vi "UHR-Fleezers Control (host) - 12.6.vi"() -> ()   [LabVIEW 2012] (continued)
          frame #0 {
            n636 = property on="Saved AOD Raster Scan Parameter Sets" class="Arr (strict)"("Index Values"=u32[] [1]) -> ()  [unwired: 2 in, 2 out]
          }
          frame #1 {
            n637 = Multiply(x="N Steps", y="Step Size (nm)") -> (x*y=w1003:dbl)
            n638 = property on="Scan Speed AOD (nm/s) 2" class="DigNum (strict)"("Value"="Step Size (nm)") -> ()  [unwired: 2 in, 2 out]
            n639 = property on="Step Size AOD (nm) 2" class="DigNum (strict)"("Value"="Step Size (nm)") -> ()  [unwired: 2 in, 2 out]
            n640 = property on="Scan Range AOD (nm) 2" class="DigNum (strict)"("Value"=w1003) -> ()  [unwired: 2 in, 2 out]
          }
        }
      }
      event "Take Detection Laser\nImage": Value Change {
        n641 = event-data() -> ()  [unwired: 1 in, 5 out]
        n642 = flat-sequence {
          tunnel: [w1031] -> w1021
          tunnel: [w1030] -> w1014
          tunnel: [w1029] -> w1006
          tunnel: [w1034] -> w1022
          tunnel: w1021 -> [w1034]
          tunnel: [w1033] -> w1015
          tunnel: w1014 -> [w1033]
          tunnel: [w1032] -> w1007
          tunnel: w1006 -> [w1032]
          tunnel: [w1038] -> w1023
          tunnel: w1022 -> [w1038]
          tunnel: [w1037] -> w1016
          tunnel: w1015 -> [w1037]
          tunnel: [w1036] -> w1008
          tunnel: w1007 -> [w1036]
          tunnel: [w1044] -> w1024
          tunnel: w1023 -> [w1044]
          tunnel: [w1043] -> w1017
          tunnel: w1016 -> [w1043]
          tunnel: [w1042] -> w1009
          tunnel: w1008 -> [w1042]
          tunnel: [w1048] -> w1025
          tunnel: w1024 -> [w1048]
          tunnel: [w1047] -> w1018
          tunnel: w1017 -> [w1047]
          tunnel: [w1046] -> w1010
          tunnel: w1009 -> [w1046]
          tunnel: [w1052] -> w1026
          tunnel: w1025 -> [w1052]
          tunnel: [w1051] -> w1019
          tunnel: w1018 -> [w1051]
          tunnel: [w1050] -> w1011
          tunnel: w1010 -> [w1050]
          tunnel: [w1056] -> w1027
          tunnel: w1026 -> [w1056]
          tunnel: [w1055] -> w1020
          tunnel: w1019 -> [w1055]
          tunnel: [w1054] -> w1012
          tunnel: w1011 -> [w1054]
          tunnel: w1027 -> [w1062]
          tunnel: w1020 -> [w1061]
          tunnel: [w1059] -> w1013
          tunnel: w1012 -> [w1059]
          tunnel: w1013 -> [w1063]
          frame #0 {
            n643 = local read "Laser interlacing mode"() -> (w1030:enum32{"Laser ON", "Laser OFF", "Interlace"})
            n644 = local read "Green FB On/Off"() -> (w1029:bool)
            n645 = local read "Green Laser ON"() -> (w1031:bool)
          }
          frame #1 {
            n646 = property on="Green FB On/Off" class="Bool (strict)"("Val(Sgnl)"=FALSE ("Value (Signaling)")) -> ()  [unwired: 2 in, 2 out]
          }
          frame #2 {
            n647 = property on="Green Laser ON" class="Bool (strict)"("Val(Sgnl)"=TRUE ("Value (Signaling)")) -> ()  [unwired: 2 in, 2 out]
            n648 = property on="Flip Green Filter" class="Bool (strict)"("Val(Sgnl)"=TRUE ("Value (Signaling)")) -> ()  [unwired: 2 in, 2 out]
            n649 = property on="Laser interlacing mode" class="RadioBtnsControl (strict)"("Val(Sgnl)"=enum32{"Laser ON", "Laser OFF", "Interlace"}."Laser ON" ("Value (Signaling)")) -> ()  [unwired: 2 in, 2 out]
          }
          frame #3 {
            n650 = Wait (ms)(milliseconds to wait=u32 500) -> ()  [unwired: 1 out]
          }
          frame #4 {
            n651 = property on="Confocal Image" class="Bool (strict)"("Val(Sgnl)"=TRUE ("Value (Signaling)")) -> ()  [unwired: 2 in, 2 out]
          }
          frame #5 {
            n652 = Wait (ms)(milliseconds to wait=u32 2000) -> ()  [unwired: 1 out]
          }
          frame #6 {
            n653 = while {
              stop <- w1057 stop-if-true
              n654 = local read "Saving..."() -> (w1058:bool)
              n655 = Not(x=w1058) -> (.not. x?=w1057:bool)
            }
          }
          frame #7 {
            n656 = property on="Flip Green Filter" class="Bool (strict)"("Val(Sgnl)"=TRUE ("Value (Signaling)")) -> ()  [unwired: 2 in, 2 out]
            n657 = property on="Green Laser ON" class="Bool (strict)"("Val(Sgnl)"=w1062) -> ()  [unwired: 2 in, 2 out]
            n658 = property on="Laser interlacing mode" class="RadioBtnsControl (strict)"("Val(Sgnl)"=w1061) -> ()  [unwired: 2 in, 2 out]
          }
          frame #8 {
            n659 = property on="Green FB On/Off" class="Bool (strict)"("Val(Sgnl)"=w1063) -> ()  [unwired: 2 in, 2 out]
          }
        }
      }
      event "Stop All": Value Change {
        # "Stopping blue laser before shutting off program"
        n660 = event-data() -> ()  [unwired: 1 in, 5 out]
        n661 = local read "Delay (ms)"() -> (w1066:i32)
        n662 = call "serial write macro.vi"("String"="l0", "Delay (ms)"=w1066, "VISA resource name"=w1069) -> ("read buffer"=w1064:string, "error out"=w1065:errorcluster, "VISA resource name out"=w1068:refnum<visa-resource-name>)
        n663 = local write "read blue buffer"(w1064) -> ()
        n664 = local write "Blue Error Out"(w1065) -> ()
        n665 = VISA Close(VISA resource name=w1068) -> ()  [unwired: 1 in, 1 out]
        n666 = local read "Stop All"() -> (w1070:bool)
      }
    }
    n667 = node-c288() -> ()  [unwired: 1 in, 1 out]
  }
  n668 = node-c288() -> (w10:T23)  [unwired: 4 out]
  n669 = timed-loop "Oscillate Trap/AOM (fishing, conjugate plane alignment)" {
    tunnel: w16 -> [w1072]
    tunnel: [w1071] -> w129
    timing: w124 -> [_]
    timing-out: [_] -> w123
    stop <- w1071 stop-if-true
    n670 = node-c288() -> ()  [unwired: 2 out]
    n671 = event shown="[0] \"Oscillate Set 1\", \"Fish for Tether\": Value Change" {
      selector: _ -> [_ _ _]
      dyn-events: _ -> [_ _ _]
      timeout: _ -> [_ _ _]
      tunnel: w1072 -> [w1079 _ _]
      tunnel: [FALSE ("Stop All") _ w1677] -> w1071
      event "Oscillate Set 1", "Fish for Tether": Value Change {
        n672 = event-data() -> ()  [unwired: 6 out]
        n673 = local read "Oscillate Set 1"() -> (w1078:bool)
        n674 = Or(x=w1078, y="Fish for Tether") -> (x .or. y?=w1076:bool)
        n675 = case shown="True" w1076 {
          tunnel: w1079 -> [_ w1082]
          tunnel: "Fish for Tether" -> [_ w1081]
          frame False {
          }
          frame True {
            n676 = case shown="True" w1081 {
              selector: w1081 -> [w1085 w1091]
              tunnel: [w1085 w1091] -> w1080
              frame False {
              }
              frame True {
                n677 = local write "Scan axis 2"(TRUE) -> ()
                n678 = local write "Tether"(FALSE ("Tether")) -> ()
                n679 = local read "Flow ON during cal?"() -> (w1086:bool)
                n680 = property on="Trap Delta (MHz)" class="DigNum (strict)"("Val(Sgnl)"="Furthest Delta (MHz)") -> ()  [unwired: 2 in, 2 out]
                n681 = Or(x="Flow ON during \nfishing?", y=w1086) -> (x .or. y?=w1087:bool)
                n682 = Wait (ms)(milliseconds to wait=u32 500) -> ()  [unwired: 1 out]
                n683 = property on="Sample Channel\nFlow" class="Bool (strict)"("Val(Sgnl)"=w1087) -> ()  [unwired: 2 in, 2 out]
              }
            }
            n684 = node-c288() -> (w1084:T23)  [unwired: 1 in, 3 out]
            n685 = timed-loop "Oscillate AOD" {
              timing: w1084 -> [_]
              timing-out: [_] -> w1083
              tunnel: w1082 -> [w1101]
              tunnel: w1080 -> [w1094]
              i -> [w1103]
              stop <- w1100 stop-if-true
              n686 = node-c288() -> (w1102:i64)  [unwired: 1 out]
              n687 = flat-sequence {
                tunnel: w1103 -> [w1130]
                tunnel: w1102 -> [w1129]
                tunnel: w1101 -> [w1111]
                tunnel: w1094 -> [w1113]
                tunnel: [w1113] -> w1099
                tunnel: [w1112] -> w1098
                tunnel: [w1110] -> w1097
                tunnel: [w1107] -> w1095
                tunnel: w1099 -> [w1175]
                tunnel: w1098 -> [w1173]
                tunnel: w1097 -> [w1172]
                tunnel: [w1171] -> w1096
                tunnel: w1095 -> [w1170]
                tunnel: [w1247] -> w1100
                tunnel: w1096 -> [w1246]
                frame #0 {
                  # "w (rad/s)"
                  # "t (s)"
                  n688 = Divide(x=w1129, y=i64 1000) -> (x/y=w1104:dbl)
                  n689 = local read "BD 1 Frequency 2 (MHz)"() -> (w1106:dbl)
                  n690 = Multiply(x="Osc. freq. (Hz)", y=6.283185307179586) -> (x*y=w1127:dbl)
                  n691 = Multiply(x=w1104, y=w1130) -> (x*y=w1126:dbl)
                  n692 = Multiply(x=w1127, y=w1126) -> (x*y=w1109:dbl)
                  n693 = local read "BD 1 Frequency 1 (MHz)"() -> (w1115:dbl)
                  n694 = case shown="True" w1113 {
                    tunnel: w1109 -> [w1136 w1153]
                    tunnel: w1115 -> [_ w1161]
                    tunnel: w1106 -> [_ w1162]
                    tunnel: [w1133 w1157] -> w1105
                    tunnel: [FALSE w1138] -> w1110
                    tunnel: [0.0 w1149] -> w1107
                    frame False {
                      n695 = Sine(x=w1136) -> (sin(x)=w1134:dbl)
                      n696 = Multiply(x=w1134, y="Osc. amp. (MHz)") -> (x*y=w1133:dbl)
                    }
                    frame True {
                      # "trap position goes from 0 to 1 (0 is when it is furthest away, 1 is when closest)\nso we want to test for tether only when farther away, or x < 1"
                      # "quit if taking too long"
                      # "oscillate the trap"
                      # "Test for tether"
                      n697 = local read "Vec Mean of T1 T2"() -> (w1137:dbl[])
                      "Trigger Signal" <- w1137
                      n698 = Cosine(x=w1153) -> (cos(x)=w1165:dbl)
                      n699 = Subtract(x=w1162, y=w1161) -> (x-y=w1160:dbl)
                      n700 = Decrement(x=w1165) -> (x-1=w1164:dbl)
                      n701 = Subtract(x=w1160, y="Closest Delta (MHz)") -> (x-y=w1158:dbl)
                      n702 = Divide(x=w1164, y=-2.0) -> (x/y=w1148:dbl)
                      n703 = Greater?(x=w1137, y="Stop F (pN)") -> (0:w1155:bool[])
                      n704 = Multiply(x=w1148, y=w1158) -> (x*y=w1157:dbl)
                      n705 = Less?(x=w1148, y="Fish mask thresh") -> (x < y?=w1147:bool)
                      n706 = Boolean To (0,1)(Boolean=w1147) -> (0, 1=w1145:i16)
                      n707 = Multiply(x=w1145, y=w1137) -> (x*y=w1144:dbl[])
                      n708 = Divide(x=w1153, y=6.283185307179586) -> (x/y=w1152:dbl)
                      n709 = Round Toward +Infinity(x=w1152) -> (ceil(x): smallest int >= x=w1149:dbl)
                      "Attempts" <- w1149
                      n710 = Greater?(x=w1144, y="Stop F (pN) (mask)") -> (0:w1142:bool[])
                      n711 = Or Array Elements(Boolean array=w1155) -> (logical OR=w1140:bool)
                      n712 = Or Array Elements(Boolean array=w1142) -> (logical OR=w1139:bool)
                      n713 = Greater?(x=w1149, y="Attempt Limit") -> (0:w1151:bool)
                      n714 = case shown="True" w1151 {
                        frame False {
                        }
                        frame True {
                          n715 = local write "Fish for Tether"(FALSE ("Fish for Tether")) -> ()
                          n716 = call <vilib>:"Beep.vi"() -> ()  [unwired: 3 in, 9 out]
                          n717 = local read "Messages"() -> (w1167:string)
                          n718 = call "Update messages.vi"("Message to add"="Tether fishing timeout." ("Messages"), "Old message string"=w1167) -> ("New message string"=→"Messages":string)
                        }
                      }
                      n719 = Select(t=w1140, s="Normal (on) or masked test (off)", f=w1139) -> (s? t:f=w1138:bool)
                    }
                  }
                  n720 = local read "BD 2 Frequency 1 (MHz)"() -> (w1114:dbl)
                  n721 = Select(t=w1115, s="Scan axis 2", f=w1114) -> (s? t:f=w1118:dbl)
                  n722 = Add(x=w1105, y=w1118) -> (x+y=w1112:dbl)
                  n723 = Select(t=w1112, s="Scan axis 2", f=w1115) -> (s? t:f=w1121:dbl)
                  n724 = Select(t=w1114, s="Scan axis 2", f=w1112) -> (s? t:f=w1120:dbl)
                  n725 = local read "BD 2 Frequency 2 (MHz)"() -> (w1123:dbl)
                  n726 = local read "BD 2 Frequency 3 (MHz)"() -> (w1122:dbl)
                  n727 = local read "Y RF Frequency Limits (MHz)"() -> (w1116:T16)
                  n728 = local read "X RF Frequency Limits (MHz)"() -> (w1117:T16)
                  n729 = local read "BD 1 Frequency 3 (MHz)"() -> (w1124:dbl)
                  n730 = call "set RF board frequency - interlace.vi"("Board 2 Frequency Limits"=w1116, "Board 1 Frequency Limits"=w1117, "FPGA VI Reference In"=w1111, "Board 2 Frequency 3 (MHz)"=w1122, "Board 1 Frequency 3 (MHz)"=w1124, "Board 2 Frequency 2 (MHz)"=w1123, "Board 2 Frequency 1 (MHz)"=w1120, "Board 1 Frequency 2 (MHz)"=w1106, "Board 1 Frequency 1  (MHz)"=w1121) -> ()  [unwired: 1 in, 2 out]
                }
                frame #1 {
                  n731 = And(x=w1175, y=w1172) -> (x .and. y?=w1174:bool)
                  n732 = case "Only if were fishing and now formed tether" shown="True" w1174 {
                    tunnel: w1173 -> [w1177 w1192]
                    tunnel: [w1176 w1191] -> w1171
                    tunnel: w1170 -> [_ w1187]
                    frame False {
                      n733 = local read "Fish for Tether"() -> (w1176:bool)
                      n734 = case shown="False" w1176 {
                        tunnel: w1177 -> [w1178 _]
                        frame False {
                          n735 = property on="BD 1 Frequency 1 (MHz)" class="DigNum (strict)"("Val(Sgnl)"=w1178) -> ()  [unwired: 2 in, 2 out]
                        }
                        frame True {
                        }
                      }
                    }
                    frame True {
                      w1191 = FALSE ("Fish for Tether")
                      n736 = call <vilib>:"Beep.vi"() -> ()  [unwired: 3 in, 9 out]
                      n737 = Number To Decimal String(number=w1187, width (-)=i16 1) -> (decimal integer string=w1185:string)
                      n738 = Concatenate Strings("Formed tether in ", w1185, " attempt(s)." ("string")) -> (w1182:string)
                      n739 = local read "Messages"() -> (w1189:string)
                      n740 = local write "Fish for Tether"(w1191) -> ()
                      n741 = call "Update messages.vi"("Message to add"=w1182, "Old message string"=w1189) -> ("New message string"=w1188:string)
                      n742 = local write "Messages"(w1188) -> ()
                      n743 = Get Date/Time In Seconds() -> (seconds since 1Jan1904=→"Time tether formed":timestamp)
                      n744 = local read "Flow ON during cal?"() -> (w1179:bool)
                      n745 = property on="Sample Channel\nFlow" class="Bool (strict)"("Val(Sgnl)"=w1179) -> (error out=w1180:errorcluster)  [unwired: 2 in, 1 out]
                      n746 = case shown="\"2\", \"3\", \"4\", \"5\", \"6\"" "Then..." {
                        selector: "Then..." -> [_ w1195]
                        tunnel: w1192 -> [w1194 _]
                        tunnel: w1180 -> [_ _]
                        frame "1", Default {
                          n747 = property on="BD 1 Frequency 1 (MHz)" class="DigNum (strict)"("Val(Sgnl)"=w1194) -> ()  [unwired: 2 in, 2 out]
                        }
                        frame "2", "3", "4", "5", "6" {
                          n748 = flat-sequence {
                            tunnel: w1195 -> [w1197]
                            frame #0 {
                              n749 = property on="Trap Delta (MHz)" class="DigNum (strict)"("Val(Sgnl)"="Move to Delta 1 (MHz)") -> ()  [unwired: 2 in, 2 out]
                            }
                            frame #1 {
                              n750 = case shown="\"5\", \"6\"" w1197 {
                                selector: w1197 -> [w1200 w1210 _]
                                frame "3", "4" {
                                n751 = flat-sequence {
                                tunnel: w1200 -> [w1201]
                                tunnel: [w1201] -> w1198
                                tunnel: [w1203] -> w1199
                                tunnel: w1198 -> [w1203]
                                tunnel: w1199 -> [w1207]
                                frame #0 {
                                n752 = property on="Green Laser ON" class="Bool (strict)"("Val(Sgnl)"=TRUE ("Value (Signaling)")) -> ()  [unwired: 2 in, 2 out]
                                }
                                frame #1 {
                                n753 = Multiply(x="Wait Before Save (s)", y=u32 1000 ("x")) -> (x*y=w1205:u32)
                                n754 = Wait (ms)(milliseconds to wait=w1205) -> ()  [unwired: 1 out]
                                }
                                frame #2 {
                                n755 = property on="Start Saving" class="Bool (strict)"("Value"=TRUE ("Start Saving")) -> ()  [unwired: 2 in, 2 out]
                                n756 = case shown="\"4\"" w1207 {
                                frame Default {
                                }
                                frame "4" {
                                n757 = property on="Fl. Triggered..." class="Bool (strict)"("Val(Sgnl)"=TRUE ("Value (Signaling)")) -> ()  [unwired: 2 in, 2 out]
                                }
                                }
                                }
                                }
                                }
                                frame "5", "6" {
                                n758 = stacked-sequence {
                                tunnel: w1210 -> [_ _ _ _ _ _ w1222]
                                frame #0 {
                                n759 = Replace Array Subset(array=u32[] [0] ("Index Values"), new element="Raster Set Upon Tether", index=0) -> (w1211:u32[])
                                n760 = property on="Saved AOD Raster Scan Parameter Sets" class="Arr (strict)"("Index Values"=w1211) -> ()  [unwired: 2 in, 2 out]
                                }
                                frame #1 {
                                n761 = Wait (ms)(milliseconds to wait=u32 500) -> ()  [unwired: 1 out]
                                }
                                frame #2 {
                                n762 = property on="Load parameters" class="Bool (strict)"("Val(Sgnl)"=TRUE ("Value (Signaling)")) -> ()  [unwired: 2 in, 2 out]
                                n763 = case shown="True" "Green ON During Raster" {
                                frame False {
                                }
                                frame True {
                                n764 = property on="Green Laser ON" class="Bool (strict)"("Val(Sgnl)"=TRUE ("Value (Signaling)")) -> ()  [unwired: 2 in, 2 out]
                                }
                                }
                                }
                                frame #3 {
                                n765 = Wait (ms)(milliseconds to wait=u32 500) -> ()  [unwired: 1 out]
                                }
                                frame #4 {
                                n766 = property on="Trap Raster Scan" class="Bool (strict)"("Val(Sgnl)"=TRUE ("Value (Signaling)")) -> ()  [unwired: 2 in, 2 out]
                                }
                                frame #5 {
                                n767 = Wait (ms)(milliseconds to wait=u32 2000) -> ()  [unwired: 1 out]
                                }
                                frame #6 {
                                n768 = flat-sequence {
                                tunnel: w1222 -> [w1229]
                                frame #0 {
                                n769 = while {
                                stop <- w1225 stop-if-true
                                n770 = local read "Raster Scanning..."() -> (w1224:bool)
                                n771 = local read "Saving..."() -> (w1227:bool)
                                n772 = Wait (ms)(milliseconds to wait=u32 100) -> ()  [unwired: 1 out]
                                n773 = Not(x=w1227) -> (.not. x?=w1226:bool)
                                n774 = Not(x=w1224) -> (.not. x?=w1223:bool)
                                n775 = And(x=w1226, y=w1223) -> (x .and. y?=w1225:bool)
                                }
                                }
                                frame #1 {
                                n776 = local read "Tether"() -> (w1230:bool)
                                n777 = case shown="True" w1230 {
                                tunnel: w1229 -> [_ w1232]
                                frame False {
                                n778 = property on="Fish for Tether" class="Bool (strict)"("Val(Sgnl)"="Fish again after \nraster break?") -> ()  [unwired: 2 in, 2 out]
                                }
                                frame True {
                                n779 = stacked-sequence {
                                tunnel: w1232 -> [_ w1236 _ _]
                                frame #0 {
                                n780 = property on="Trap Delta (MHz)" class="DigNum (strict)"("Val(Sgnl)"="Move to Delta 2 (MHz)") -> ()  [unwired: 2 in, 2 out]
                                n781 = case shown="True" "Flow ON after\ntether testing?" {
                                frame False {
                                }
                                frame True {
                                n782 = property on="Sample Channel\nFlow" class="Bool (strict)"("Val(Sgnl)"=TRUE ("Value (Signaling)")) -> ()  [unwired: 2 in, 2 out]
                                }
                                }
                                }
                                frame #1 {
                                n783 = flat-sequence {
                                tunnel: w1236 -> [w1238]
                                frame #0 {
                                n784 = Wait (ms)(milliseconds to wait=u32 500) -> ()  [unwired: 1 out]
                                }
                                frame #1 {
                                n785 = case shown="\"6\"" w1238 {
                                frame Default {
                                }
                                frame "6" {
                                n786 = property on="Green Laser ON" class="Bool (strict)"("Val(Sgnl)"=TRUE ("Green Laser ON/Interlacing")) -> ()  [unwired: 2 in, 2 out]
                                }
                                }
                                }
                                frame #2 {
                                n787 = Wait (ms)(milliseconds to wait=u32 500) -> ()  [unwired: 1 out]
                                }
                                frame #3 {
                                n788 = local write "Start Saving"("Save at end (5, 6)") -> ()
                                }
                                }
                                }
                                frame #2 {
                                n789 = local read "Bead Sep. Int. Time (s)"() -> (w1244:dbl)
                                n790 = Multiply(x=w1244, y=1000.0) -> (x*y=w1243:dbl)
                                n791 = Wait (ms)(milliseconds to wait=w1243) -> ()  [unwired: 1 out]
                                }
                                frame #3 {
                                n792 = property on="Remove Offset" class="Bool (strict)"("Val(Sgnl)"=TRUE ("Value (Signaling)")) -> ()  [unwired: 2 in, 2 out]
                                }
                                }
                                }
                                }
                                }
                                }
                                }
                                }
                                }
                                frame "2", Default {
                                }
                              }
                            }
                          }
                        }
                      }
                      "Tether" <- "Tether Alarm?"
                    }
                  }
                }
                frame #2 {
                  n793 = local read "Oscillate Set 1"() -> (w1251:bool)
                  n794 = local read "Stop All"() -> (w1249:bool)
                  n795 = Or(x=w1251, y=w1246) -> (x .or. y?=w1248:bool)
                  n796 = Not(x=w1248) -> (.not. x?=w1250:bool)
                  n797 = Compound Arithmetic op=OR(w1249, w1250) -> (w1247:bool)
                }
              }
              n798 = node-c288() -> ()  [unwired: 2 out]
            }
            n799 = node-c288(w1083) -> ()  [unwired: 1 out]
          }
        }
      }
      event "Fl. Triggered...": Value Change {
        n800 = event-data() -> ()  [unwired: 7 out]
        n801 = case shown="True" "Fl. Triggered..." {
          frame False {
          }
          frame True {
            n802 = node-c288() -> (w1262:T23)  [unwired: 4 out]
            n803 = timed-loop {
              timing: w1262 -> [_]
              timing-out: [_] -> w1261
              tunnel: "Action" -> [w1270]
              shift-right: [w1267] -> _
              shift-left: u8 255 -> [w1269]
              shift-right: [w1264] -> _
              shift-left: 255 -> [w1266]
              stop <- w1263 stop-if-true
              # "Reset confocal spot"
              n804 = node-c288() -> ()  [unwired: 2 out]
              n805 = flat-sequence {
                tunnel: w1270 -> [w1290]
                tunnel: w1269 -> [w1289]
                tunnel: [w1288] -> w1268
                tunnel: w1266 -> [w1275]
                tunnel: [w1274] -> w1265
                tunnel: [w1669] -> w1263
                tunnel: w1268 -> [w1668]
                tunnel: [w1668] -> w1267
                tunnel: [w1667] -> w1264
                tunnel: w1265 -> [w1667]
                frame #0 {
                  n806 = local read "Delta Fl. 2"() -> (w1287:dbl)
                  n807 = local read "Delta Fl. 1"() -> (w1282:dbl)
                  n808 = Multiply(x="Fl. Delta Thresh. (kHz)", y=1000.0) -> (x*y=w1277:dbl)
                  n809 = Select(t=w1282, s="APD to Watch", f=w1287) -> (s? t:f=w1278:dbl)
                  n810 = Greater?(x=w1278, y=w1277) -> (0:w1283:bool)
                  n811 = Or(x="Force Yank", y=w1283) -> (x .or. y?=w1281:bool)
                  n812 = And(x=w1281, y="Yank when?") -> (x .and. y?=w1279:bool)
                  n813 = case shown="False" w1279 {
                    tunnel: w1290 -> [w1293 w1494]
                    tunnel: w1289 -> [w1295 w1490]
                    tunnel: [w1295 w1488] -> w1288
                    tunnel: w1278 -> [w1301 _]
                    tunnel: w1277 -> [w1300 _]
                    tunnel: "Force Yank" -> [w1298 _]
                    tunnel: w1275 -> [w1297 w1487]
                    tunnel: [w1296 w1487] -> w1274
                    frame False {
                      n814 = Negate(x=w1300) -> (-x=w1292:dbl)
                      n815 = local write "Fl. High"(TRUE ("Fl. High")) -> ()
                      n816 = Less?(x=w1301, y=w1292) -> (x < y?=w1299:bool)
                      n817 = Or(x=w1298, y=w1299) -> (x .or. y?=w1294:bool)
                      n818 = case shown="True" w1294 {
                        tunnel: w1297 -> [w1302 w1312]
                        tunnel: [w1302 w1311] -> w1296
                        tunnel: w1293 -> [_ w1310]
                        frame False {
                        }
                        frame True {
                          n819 = flat-sequence {
                            tunnel: w1312 -> [w1318]
                            tunnel: w1310 -> [w1315]
                            tunnel: [w1317] -> w1309
                            tunnel: [w1316] -> w1308
                            tunnel: [w1315] -> w1307
                            tunnel: w1306 -> [w1314]
                            tunnel: [w1314] -> w1305
                            tunnel: w1304 -> [w1313]
                            tunnel: [w1313] -> w1303
                            tunnel: [w1389] -> w1311
                            tunnel: w1309 -> [w1389]
                            tunnel: w1308 -> [w1388]
                            tunnel: w1307 -> [w1387]
                            tunnel: w1305 -> [w1386]
                            tunnel: w1303 -> [w1385]
                            frame #0 {
                              n820 = call <vilib>:"Beep.vi"() -> ()  [unwired: 12 in]
                              n821 = local write "Waiting"(FALSE ("Waiting")) -> ()
                              n822 = Increment(x=w1318) -> (x+1=w1317:i32)
                              n823 = case shown="\"Image\"" w1315 {
                                tunnel: w1317 -> [_ w1323 _]
                                frame "Alarm", Default {
                                }
                                frame "Yank" {
                                n824 = flat-sequence {
                                tunnel: w1323 -> [w1326]
                                tunnel: [w1325] -> w1322
                                tunnel: [w1324] -> w1321
                                tunnel: w1322 -> [w1336]
                                tunnel: w1321 -> [w1337]
                                frame #0 {
                                n825 = local read "Yank Delay (s)"() -> (w1329:dbl)
                                n826 = local read "N Array El"() -> (w1324:u8)
                                n827 = Quotient & Remainder(x=w1326, y=w1324) -> (x-y*floor(x/y)=w1325:i32)  [unwired: 1 out]
                                n828 = Multiply(x=w1329, y=1000.0) -> (x*y=w1327:dbl)
                                n829 = Wait (ms)(milliseconds to wait=w1327) -> ()  [unwired: 1 out]
                                }
                                frame #1 {
                                n830 = local read "Yank to which?"() -> (w1331:bool)
                                n831 = local read "Random Choice"() -> (w1341:bool)
                                n832 = local read "Yank to Trap Delta (MHz)"() -> (w1334:dbl[])
                                n833 = local read "Yank to SP"() -> (w1335:dbl[])
                                n834 = Random Number (0-1)() -> (number: 0 to 1=w1340:dbl)
                                n835 = Multiply(x=w1337, y=w1340) -> (x*y=w1339:dbl)
                                n836 = Round Toward -Infinity(1:w1339) -> (0:w1338:dbl)
                                n837 = Select(t=w1338, s=w1341, f=w1336) -> (s? t:f=w1332:dbl)
                                n838 = Select(t=w1334, s=w1331, f=w1335) -> (s? t:f=w1333:dbl[])
                                n839 = Index Array(array=w1333, index=w1332) -> (element=w1330:dbl)
                                n840 = case shown="True" w1331 {
                                tunnel: w1330 -> [w1342 w1369]
                                frame False {
                                n841 = flat-sequence {
                                tunnel: w1342 -> [w1343]
                                frame #0 {
                                n842 = property on="Trap Pos FB SP" class="DigNum (strict)"("Val(Sgnl)"=w1343) -> ()  [unwired: 2 in, 2 out]
                                }
                                frame #1 {
                                n843 = Wait (ms)(milliseconds to wait=u32 700) -> ()  [unwired: 1 out]
                                }
                                frame #2 {
                                n844 = local read "Action (%)"() -> (w1348:dbl)
                                n845 = Absolute Value(x=w1348) -> (abs(x)=w1347:dbl)
                                n846 = Greater?(x=w1347, y=70.0) -> (0:w1345:bool)
                                n847 = property on="Remove Action Offset" class="Bool (strict)"("Val(Sgnl)"=w1345) -> ()  [unwired: 2 in, 2 out]
                                }
                                frame #3 {
                                n848 = for {
                                N: 4 -> [_]
                                n849 = flat-sequence {
                                frame #0 {
                                n850 = Wait (ms)(milliseconds to wait=u32 500) -> ()  [unwired: 1 out]
                                }
                                frame #1 {
                                n851 = local read "Action (%)"() -> (w1354:dbl)
                                n852 = Absolute Value(x=w1354) -> (abs(x)=w1353:dbl)
                                n853 = Greater?(x=w1353, y=70.0) -> (0:w1351:bool)
                                n854 = property on="Remove Action Offset" class="Bool (strict)"("Val(Sgnl)"=w1351) -> ()  [unwired: 2 in, 2 out]
                                }
                                }
                                }
                                }
                                frame #4 {
                                n855 = Wait (ms)(milliseconds to wait=u32 500) -> ()  [unwired: 1 out]
                                }
                                frame #5 {
                                n856 = local read "Mean"() -> (w1362:dbl)
                                n857 = Greater?(x=w1362, y=11.0) -> (0:w1356:bool)
                                n858 = Not(x=w1356) -> (.not. x?=w1357:bool)
                                n859 = And(x=w1357, y="Shift confocal") -> (x .and. y?=w1359:bool)
                                n860 = And(x=w1356, y="Shift confocal") -> (x .and. y?=w1360:bool)
                                n861 = case shown="True" w1360 {
                                frame False {
                                }
                                frame True {
                                n862 = local read "Confocal Y 2 (V)"() -> (w1366:dbl)
                                n863 = local read "Confocal X 2 (V)"() -> (w1365:dbl)
                                n864 = property on="AO1" class="Slide (strict)"("Val(Sgnl)"=w1366) -> ()  [unwired: 2 in, 2 out]
                                n865 = property on="AO2" class="Slide (strict)"("Val(Sgnl)"=w1365) -> ()  [unwired: 2 in, 2 out]
                                }
                                }
                                n866 = case shown="True" w1359 {
                                frame False {
                                }
                                frame True {
                                n867 = local read "Confocal Y 1 (V)"() -> (w1364:dbl)
                                n868 = local read "Confocal X 1 (V)"() -> (w1363:dbl)
                                n869 = property on="AO1" class="Slide (strict)"("Val(Sgnl)"=w1364) -> ()  [unwired: 2 in, 2 out]
                                n870 = property on="AO2" class="Slide (strict)"("Val(Sgnl)"=w1363) -> ()  [unwired: 2 in, 2 out]
                                }
                                }
                                }
                                frame #6 {
                                n871 = Wait (ms)(milliseconds to wait=u32 1500) -> ()  [unwired: 1 out]
                                }
                                frame #7 {
                                n872 = property on="Rem fb disp offset" class="Bool (strict)"("Val(Sgnl)"=TRUE ("Value (Signaling)")) -> ()  [unwired: 2 in, 2 out]
                                }
                                }
                                }
                                frame True {
                                n873 = flat-sequence {
                                tunnel: w1369 -> [w1370]
                                frame #0 {
                                n874 = property on="Trap Delta (MHz)" class="DigNum (strict)"("Val(Sgnl)"=w1370) -> ()  [unwired: 2 in, 2 out]
                                }
                                frame #1 {
                                n875 = Wait (ms)(milliseconds to wait=u32 500) -> ()  [unwired: 1 out]
                                }
                                frame #2 {
                                n876 = local read "Shift confocal"() -> (w1376:bool)
                                n877 = local read "Mean"() -> (w1378:dbl)
                                n878 = Greater?(x=w1378, y=11.0) -> (0:w1375:bool)
                                n879 = Not(x=w1375) -> (.not. x?=w1374:bool)
                                n880 = And(x=w1374, y=w1376) -> (x .and. y?=w1372:bool)
                                n881 = And(x=w1375, y=w1376) -> (x .and. y?=w1373:bool)
                                n882 = case shown="True" w1373 {
                                frame False {
                                }
                                frame True {
                                n883 = local read "Confocal Y 2 (V)"() -> (w1382:dbl)
                                n884 = local read "Confocal X 2 (V)"() -> (w1381:dbl)
                                n885 = property on="AO2" class="Slide (strict)"("Val(Sgnl)"=w1381) -> ()  [unwired: 2 in, 2 out]
                                n886 = property on="AO1" class="Slide (strict)"("Val(Sgnl)"=w1382) -> ()  [unwired: 2 in, 2 out]
                                }
                                }
                                n887 = case shown="True" w1372 {
                                frame False {
                                }
                                frame True {
                                n888 = local read "Confocal X 1 (V)"() -> (w1379:dbl)
                                n889 = local read "Confocal Y 1 (V)"() -> (w1380:dbl)
                                n890 = property on="AO2" class="Slide (strict)"("Val(Sgnl)"=w1379) -> ()  [unwired: 2 in, 2 out]
                                n891 = property on="AO1" class="Slide (strict)"("Val(Sgnl)"=w1380) -> ()  [unwired: 2 in, 2 out]
                                }
                                }
                                }
                                }
                                }
                                }
                                }
                                }
                                }
                                frame "Image" {
                                n892 = property on="Confocal Image" class="Bool (strict)"("Val(Sgnl)"=TRUE ("Value (Signaling)")) -> ()  [unwired: 2 in, 2 out]
                                }
                              }
                              n893 = local write "Fl. High"(FALSE ("Fl. High")) -> ()
                              n894 = local read "Time (s)"() -> (w1316:dbl)
                            }
                            frame #1 {
                              n895 = case shown="True" "Auto F Reset" {
                                tunnel: w1388 -> [_ w1393]
                                tunnel: w1387 -> [_ w1392]
                                tunnel: w1386 -> [_ w1391]
                                tunnel: w1385 -> [_ w1390]
                                frame False {
                                }
                                frame True {
                                n896 = node-c288() -> (w1395:T23)  [unwired: 4 in]
                                n897 = timed-loop {
                                timing: w1395 -> [_]
                                timing-out: [_] -> w1394
                                tunnel: w1393 -> [w1400]
                                tunnel: w1392 -> [w1399]
                                tunnel: w1391 -> [w1398]
                                tunnel: w1390 -> [w1397]
                                stop <- w1396 stop-if-true
                                n898 = node-c288() -> ()  [unwired: 1 in, 1 out]
                                n899 = local read "Fl. Delta Thresh. (kHz)"() -> (w1409:dbl)
                                n900 = local read "APD to Watch"() -> (w1410:bool)
                                n901 = local read "Delta Fl. 1"() -> (w1411:dbl)
                                n902 = local read "Delta Fl. 2"() -> (w1412:dbl)
                                n903 = local read "Fl. Triggered..."() -> (w1403:bool)
                                n904 = local read "Stop All"() -> (w1404:bool)
                                n905 = local read "Reset Force"() -> (w1402:bool)
                                n906 = Multiply(x=w1409, y=1000.0) -> (x*y=w1407:dbl)
                                n907 = Select(t=w1411, s=w1410, f=w1412) -> (s? t:f=w1406:dbl)
                                n908 = Not(x=w1403) -> (.not. x?=w1401:bool)
                                n909 = Greater?(x=w1406, y=w1407) -> (0:w1405:bool)
                                n910 = Compound Arithmetic op=OR(w1405, w1404, w1401, w1402) -> (w1396:bool)
                                n911 = case shown="True" w1396 {
                                tunnel: w1400 -> [_ w1416]
                                tunnel: w1399 -> [_ w1420]
                                tunnel: w1398 -> [_ w1419]
                                tunnel: w1397 -> [_ w1418]
                                frame False {
                                }
                                frame True {
                                n912 = case shown="\"Yank\"" w1420 {
                                tunnel: w1419 -> [_ w1430]
                                tunnel: w1418 -> [_ w1428]
                                frame "Image", Default {
                                }
                                frame "Yank" {
                                n913 = flat-sequence {
                                tunnel: [w1433] -> w1431
                                tunnel: w1430 -> [w1433]
                                tunnel: [w1432] -> w1429
                                tunnel: w1428 -> [w1432]
                                tunnel: w1431 -> [w1439]
                                tunnel: w1429 -> [w1437]
                                frame #0 {
                                n914 = local read "Yank Delay (s)"() -> (w1436:dbl)
                                n915 = Multiply(x=w1436, y=1000.0) -> (x*y=w1434:dbl)
                                n916 = Wait (ms)(milliseconds to wait=w1434) -> ()  [unwired: 1 out]
                                }
                                frame #1 {
                                n917 = local read "Yank to which?"() -> (w1438:bool)
                                n918 = case shown="False" w1438 {
                                tunnel: w1439 -> [_ w1467]
                                tunnel: w1437 -> [w1440 _]
                                frame False {
                                n919 = flat-sequence {
                                tunnel: w1440 -> [w1441]
                                frame #0 {
                                n920 = property on="Trap Pos FB SP" class="DigNum (strict)"("Val(Sgnl)"=w1441) -> ()  [unwired: 2 in, 2 out]
                                }
                                frame #1 {
                                n921 = Wait (ms)(milliseconds to wait=u32 700) -> ()  [unwired: 1 out]
                                }
                                frame #2 {
                                n922 = local read "Action (%)"() -> (w1446:dbl)
                                n923 = Absolute Value(x=w1446) -> (abs(x)=w1445:dbl)
                                n924 = Greater?(x=w1445, y=70.0) -> (0:w1443:bool)
                                n925 = property on="Remove Action Offset" class="Bool (strict)"("Val(Sgnl)"=w1443) -> ()  [unwired: 2 in, 2 out]
                                }
                                frame #3 {
                                n926 = for {
                                N: 4 -> [_]
                                n927 = flat-sequence {
                                frame #0 {
                                n928 = Wait (ms)(milliseconds to wait=u32 500) -> ()  [unwired: 1 out]
                                }
                                frame #1 {
                                n929 = local read "Action (%)"() -> (w1452:dbl)
                                n930 = Absolute Value(x=w1452) -> (abs(x)=w1451:dbl)
                                n931 = Greater?(x=w1451, y=70.0) -> (0:w1449:bool)
                                n932 = property on="Remove Action Offset" class="Bool (strict)"("Val(Sgnl)"=w1449) -> ()  [unwired: 2 in, 2 out]
                                }
                                }
                                }
                                }
                                frame #4 {
                                n933 = Wait (ms)(milliseconds to wait=u32 500) -> ()  [unwired: 1 out]
                                }
                                frame #5 {
                                n934 = local read "Shift confocal"() -> (w1457:bool)
                                n935 = local read "Mean"() -> (w1460:dbl)
                                n936 = Greater?(x=w1460, y=11.0) -> (0:w1456:bool)
                                n937 = Not(x=w1456) -> (.not. x?=w1455:bool)
                                n938 = And(x=w1456, y=w1457) -> (x .and. y?=w1458:bool)
                                n939 = And(x=w1455, y=w1457) -> (x .and. y?=w1454:bool)
                                n940 = case shown="True" w1458 {
                                frame False {
                                }
                                frame True {
                                n941 = local read "Confocal X 2 (V)"() -> (w1463:dbl)
                                n942 = local read "Confocal Y 2 (V)"() -> (w1464:dbl)
                                n943 = property on="AO2" class="Slide (strict)"("Val(Sgnl)"=w1463) -> ()  [unwired: 2 in, 2 out]
                                n944 = property on="AO1" class="Slide (strict)"("Val(Sgnl)"=w1464) -> ()  [unwired: 2 in, 2 out]
                                }
                                }
                                n945 = case shown="True" w1454 {
                                frame False {
                                }
                                frame True {
                                n946 = local read "Confocal Y 1 (V)"() -> (w1462:dbl)
                                n947 = local read "Confocal X 1 (V)"() -> (w1461:dbl)
                                n948 = property on="AO1" class="Slide (strict)"("Val(Sgnl)"=w1462) -> ()  [unwired: 2 in, 2 out]
                                n949 = property on="AO2" class="Slide (strict)"("Val(Sgnl)"=w1461) -> ()  [unwired: 2 in, 2 out]
                                }
                                }
                                }
                                frame #6 {
                                n950 = Wait (ms)(milliseconds to wait=u32 1500) -> ()  [unwired: 1 out]
                                }
                                frame #7 {
                                n951 = property on="Rem fb disp offset" class="Bool (strict)"("Val(Sgnl)"=TRUE ("Value (Signaling)")) -> ()  [unwired: 2 in, 2 out]
                                }
                                }
                                }
                                frame True {
                                n952 = flat-sequence {
                                tunnel: w1467 -> [w1468]
                                frame #0 {
                                n953 = property on="Trap Delta (MHz)" class="DigNum (strict)"("Val(Sgnl)"=w1468) -> ()  [unwired: 2 in, 2 out]
                                }
                                frame #1 {
                                n954 = Wait (ms)(milliseconds to wait=u32 500) -> ()  [unwired: 1 out]
                                }
                                frame #2 {
                                n955 = local read "Shift confocal"() -> (w1474:bool)
                                n956 = local read "Mean"() -> (w1475:dbl)
                                n957 = Greater?(x=w1475, y=11.0) -> (0:w1473:bool)
                                n958 = And(x=w1473, y=w1474) -> (x .and. y?=w1471:bool)
                                n959 = Not(x=w1473) -> (.not. x?=w1472:bool)
                                n960 = And(x=w1472, y=w1474) -> (x .and. y?=w1470:bool)
                                n961 = case shown="True" w1471 {
                                frame False {
                                }
                                frame True {
                                n962 = local read "Confocal Y 2 (V)"() -> (w1480:dbl)
                                n963 = local read "Confocal X 2 (V)"() -> (w1479:dbl)
                                n964 = property on="AO1" class="Slide (strict)"("Val(Sgnl)"=w1480) -> ()  [unwired: 2 in, 2 out]
                                n965 = property on="AO2" class="Slide (strict)"("Val(Sgnl)"=w1479) -> ()  [unwired: 2 in, 2 out]
                                }
                                }
                                n966 = case shown="True" w1470 {
                                frame False {
                                }
                                frame True {
                                n967 = local read "Confocal Y 1 (V)"() -> (w1478:dbl)
                                n968 = local read "Confocal X 1 (V)"() -> (w1477:dbl)
                                n969 = property on="AO2" class="Slide (strict)"("Val(Sgnl)"=w1477) -> ()  [unwired: 2 in, 2 out]
                                n970 = property on="AO1" class="Slide (strict)"("Val(Sgnl)"=w1478) -> ()  [unwired: 2 in, 2 out]
                                }
                                }
                                }
                                }
                                }
                                }
                                }
                                }
                                }
                                }
                                n971 = local read "Time (s)"() -> (w1415:dbl)
                                n972 = Subtract(x=w1416, y=w1415) -> (x-y=w1427:dbl)
                                n973 = Number To Decimal String(number=w1427, width (-)=i16 0) -> (decimal integer string=w1425:string)
                                n974 = Concatenate Strings(w1425, " s fluorescence event") -> (w1422:string)
                                n975 = local read "Messages"() -> (w1423:string)
                                n976 = local write "Duration (s)"(w1427) -> ()
                                n977 = call "Update messages.vi"("Message to add"=w1422, "Old message string"=w1423) -> ("New message string"=w1421:string)
                                n978 = local write "Messages"(w1421) -> ()
                                n979 = call <vilib>:"Beep.vi"() -> ()  [unwired: 12 in]
                                n980 = local write "Reset Force"(FALSE ("Force Reset")) -> ()
                                n981 = local write "Fl. High"(TRUE ("Fl. High")) -> ()
                                n982 = local write "Waiting"(TRUE ("Waiting")) -> ()
                                }
                                }
                                n983 = node-c288() -> ()  [unwired: 1 in, 1 out]
                                }
                                n984 = node-c288(w1394) -> ()  [unwired: 1 out]
                                }
                              }
                            }
                          }
                          n985 = local read "Trap Delta (MHz)"() -> (w1306:dbl)
                          n986 = local read "Trap Pos FB SP"() -> (w1304:fxp<+/-,16,1>)
                        }
                      }
                    }
                    frame True {
                      n987 = flat-sequence {
                        tunnel: w1491 -> [w1501]
                        tunnel: [w1501] -> w1495
                        tunnel: w1494 -> [w1500]
                        tunnel: [w1500] -> w1493
                        tunnel: [w1499] -> w1492
                        tunnel: w1490 -> [w1498]
                        tunnel: [w1497] -> w1489
                        tunnel: w1486 -> [w1496]
                        tunnel: [w1496] -> w1485
                        tunnel: w1495 -> [w1571]
                        tunnel: w1493 -> [w1570]
                        tunnel: w1492 -> [w1569]
                        tunnel: w1489 -> [w1568]
                        tunnel: w1485 -> [w1567]
                        tunnel: [w1568] -> w1488
                        frame #0 {
